vi "Read Attributes.vi"(11 "Create Room Service Request Msg":refnum<class "Create Room Service Request Msg.lvclass">) -> (2 "Payload":T1)   [LabVIEW 2023, in "Room Service Manager UI.lvlib" / "Create Room Service Request Msg.lvclass"]
uses:
  Create Room Service Request Msg.lvclass
  Create Room Service Request Msg.lvclass/Create Room Service Request Msg.ctl
  Room Service Types/Room Service Base/Room Service Base.lvclass
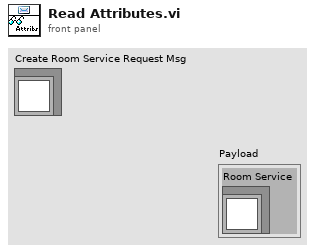
[diagram p1: front panel]
types:
  T1 = cluster{"Room Service":refnum<class "Room Service Base.lvclass">}
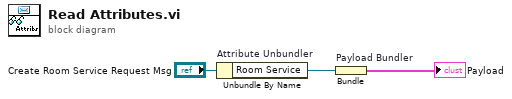
[diagram p0: block diagram]
diagram:
  n1 = Unbundle By Name "Attribute Unbundler"("Create Room Service Request Msg") -> ("Room Service"=w1:refnum<class "Room Service Base.lvclass">)
  n2 = Bundle "Payload Bundler"("Room Service"=w1) -> (→"Payload":T1)  [unwired: 1 in]
